vi "core_path_to_wait_for_notification.vi"() -> (0 "path to vi":path)   [LabVIEW 2015]
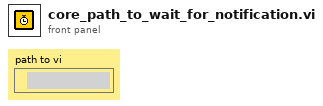
[diagram p1: front panel]
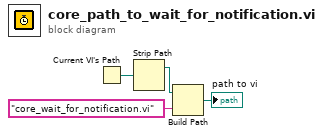
[diagram p0: block diagram]
diagram:
  n1 = Current VI's Path() -> (path=w1:path)
  n2 = Strip Path(path=w1) -> (stripped path=w4:path)  [unwired: 1 out]
  n3 = Build Path(base path=w4, name or relative path="core_wait_for_notification.vi") -> (appended path=→"path to vi":path)
